vi "Reverse triangle (for interior regions).vi"(1 "Triangle in":T1) -> (0 "Triangle out":T1)   [LabVIEW 2014]
uses:
  Typedefs/Triangle.ctl
panel:
  # "PN 13/01/2015"
  # "Vertices"
  # "Edges"
  # "Unit normal"
  # "pre-store"
  # "Vertices"
  # "Edges"
  # "Unit normal"
  # "pre-store"
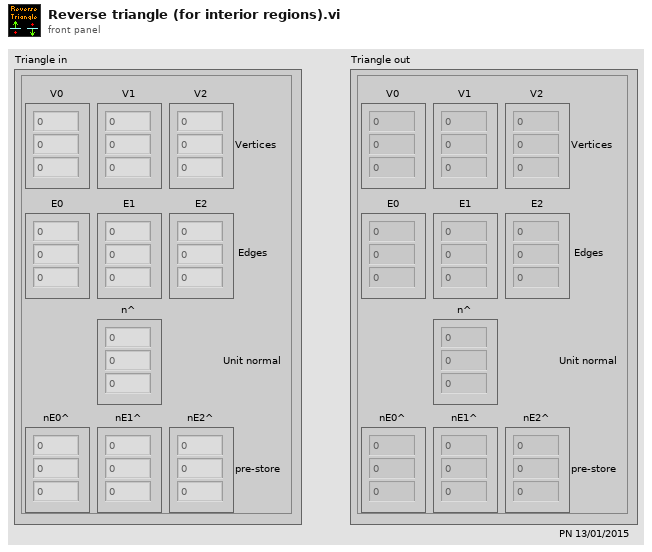
[diagram p1: front panel]
types:
  T1 = typedef "Triangle.ctl" = cluster{"V0":sgl[], "V1":sgl[], "V2":sgl[], "E0":sgl[], "E1":sgl[], "E2":sgl[], "n^":sgl[], "nE0^":sgl[], "nE1^":sgl[], "nE2^":sgl[]}
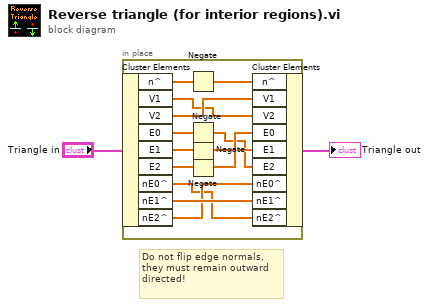
[diagram p0: block diagram]
diagram:
  # "Do not flip edge normals, they must remain outward directed!"
  n1 = in-place {
    n2 = in-place-cluster #1("Triangle in") -> ("n^"=w15:sgl[], "V1"=w9:sgl[], "V2"=w10:sgl[], "E0"=w13:sgl[], "E1"=w12:sgl[], "E2"=w11:sgl[], "nE0^"=w3:sgl[], "nE1^"=w5:sgl[], "nE2^"=w4:sgl[])
    n3 = Negate(x=w15) -> (-x=w14:sgl[])
    n4 = Negate(x=w13) -> (-x=w6:sgl[])
    n5 = Negate(x=w12) -> (-x=w7:sgl[])
    n6 = Negate(x=w11) -> (-x=w8:sgl[])
    n7 = in-place-cluster #1("n^"=w14, "V1"=w10, "V2"=w9, "E0"=w8, "E1"=w7, "E2"=w6, "nE0^"=w4, "nE1^"=w5, "nE2^"=w3) -> (→"Triangle out":T1)
  }
